vi "Check PassWord.vi"(8 "error in (no error)":errorcluster, 9 "Permission":T1, 10 "Caller ActorQName":string, 11 "CheckPasswordUI in":refnum<class "CheckPasswordUI.lvclass">) -> (0 "error out":errorcluster, 3 "CheckPasswordUI out":refnum<class "CheckPasswordUI.lvclass">)   [LabVIEW 2021, in "CheckPasswordUI.lvclass"]
uses:
  CheckPasswordUI.lvclass
  <vilib>/ActorFramework/Actor/Actor.lvclass
  <userlib>/John_Lib/Interfaces/InsertRightSubPanel/InsertRightSubPanel Messages/Insert Right SubPanel Msg/Insert Right SubPanel Msg.lvclass
  C:/Program Files (x86)/National Instruments/LabVIEW 2021/user.lib/John_Lib/AbstractActorTemplate/AbstractActorTemplate/UIActorTop.lvclass
  C:/Program Files (x86)/National Instruments/LabVIEW 2021/vi.lib/ActorFramework/Actor/Actor.lvclass
  C:/Program Files (x86)/National Instruments/LabVIEW 2021/project/Create Actor from Template/_CheckPasswordUI/CheckPasswordUI.lvclass
  C:/Program Files (x86)/National Instruments/LabVIEW 2021/user.lib/John_Lib/Interfaces/CheckPassWord/CheckPassWord.lvclass
  C:/Program Files (x86)/National Instruments/LabVIEW 2021/user.lib/John_Lib/Interfaces/InsertSubPanel/InsertSubPanel.lvclass
  <userlib>/John_Lib/Interfaces/CheckPassWord/Permission.ctl
  <userlib>/John_Lib/Interfaces/CheckPassWord/CheckPassWord.lvclass
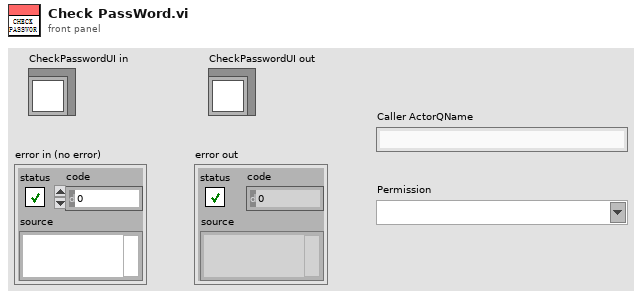
[diagram p1: front panel]
types:
  T1 = typedef "CheckPassWord.lvlib/CheckPassWord.lvclass/Permission.ctl" = string
  T2 = typedef "CheckPasswordUI.lvclass/DVR.ctl" = cluster{"Caller ActorQName":string, "Permission":T1, "PermissionNum":i32}
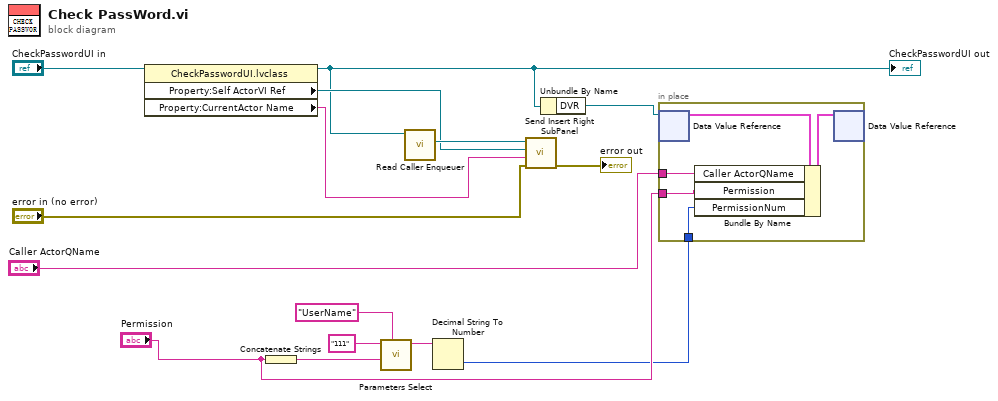
[diagram p0: block diagram]
diagram:
  n1 = property class="CheckPasswordUI.lvclass"(reference="CheckPasswordUI in") -> (reference out=w7:refnum<class "CheckPasswordUI.lvclass">, "Property:Self ActorVI Ref"=w13:refnum<vi>, "Property:CurrentActor Name"=w15:string)  [unwired: 1 in, 1 out]
  "CheckPasswordUI out" <- w7
  n2 = Concatenate Strings("Permission") -> (w6:string)
  n3 = call <userlib>:"Parameters Select.vi"("Main"="UserName", "VariableName"=w6, "Sub"="111") -> ("Value1"=w5:string)  [unwired: 4 in, 4 out]
  n4 = call <vilib>:"Read Caller Enqueuer.vi"("Actor"=w7) -> ("Caller Enqueuer"=w14:refnum<class "Message Enqueuer.lvclass">)  [unwired: 10 in]
  n5 = Decimal String To Number(string=w5) -> (number=w1:i32)  [unwired: 2 in, 1 out]
  n6 = call <userlib>:"Send Insert Right SubPanel.vi"("error in (no error)"="error in (no error)", "ActorQName"=w15, "ActorVI Ref"=w13, "Message Enqueuer"=w14) -> ("error out"=→"error out":errorcluster)  [unwired: 6 in, 1 out]
  n7 = Unbundle By Name(w7) -> ("DVR"=w9:refnum<data-value>)
  n8 = in-place {
    in-place-border: "Caller ActorQName" -> [w18]
    in-place-border: "Permission" -> [w17]
    in-place-border: w1 -> [w16]
    n9 = in-place-dvr #1(w9) -> (w20:T2)  [unwired: 1 out]
    n10 = Bundle By Name(cluster=w20, "Caller ActorQName"=w18, "Permission"=w17, "PermissionNum"=w16) -> (w19:T2)
    n11 = in-place-dvr #1(w19) -> ()  [unwired: 2 out]
  }
